vi "Set Echo Trigger Mode [ETM].vi"(7 "Micropulse # In":i32, 8 "error in (no error)":errorcluster, 9 "ETM Mode":T1, 11 "Test Number":u32) -> (0 "error out":errorcluster, 5 "Micropulse # Out":i32)   [LabVIEW 2026, in "MicroPulse_Driver.lvlib"]
doc: "Selects/deselects Interface Echo Trigger Modes, sometimes referred to as immersion testing with echo start. There several modes, one for calibration in conventional tests, one for echo trigger inspection in conventional/Phased Array tests and one for echo gate inspection in FMC tests. In echo trigger modes the echo gate is specified by the EGT(S) command and the inspection gate by the IGT(S) command. The trigger threshold level of the interface echo is set by the EUPL command for conventional tests and the EPL(S) command for Phased Array tests.\n\nMode = 0 : Normal triggering. (Default)\nMode = 1 : Display mode forms part of the calibration for conventional tests. Only the ‘Echo Gate’ is displayed allowing precise adjustment via the ‘EGT’ command.\n\nMode = 2 : Echo Trigger Mode for conventional tests. If a signal above the EUPL (is detected within the echo gate (EGT), MicroPulse processes the part of the signal derived from the IGT Parameters taken relative to the point in the echo gate where the signal breaks the EUPL.\n\nMode = 3 : For FMC Tests (AMP modes 13):\nEcho Trigger Mode for FMC tests If a signal above the EPL is detected within the echo gate (EGT), MicroPulse processes the part of the signal derived from the IGT Parameters taken relative to the point in the echo gate where the signal breaks the EPL. This happens independently on each receive channel used in the law. The data messages use a universal header format to accommodate the extra information required in this mode. For details on FMC mode interface echo see Appendix 6.5\nFor Multi-gate Tests (AMP modes 31 & 32):\nThe system performs interface echo mode and also output an Ascan that is referenced to the initial trigger. The interface echo range is now reported. It is now possible to set up an interface trigger gate, 4 hardware peak detection gates and 1 Ascan data gate on the same test. The interface echo range is output in an EGT range message (see Output Messages section)\n\nMode = 4 : Reserved\n\nMode = 5 : Echo Trigger Mode for Phased Array tests where a channel a contained within the focal law is specified as the interface trigger channel. The trigger channel must be contained within the focal law of the test. If a new focal law is applied to a test then the ETM mode is set back to 0, so the ETM mode (and therefore the trigger channel) must be resent. The interface echo range is output in an EGT range message (see Output messages section).\n\nParameters:\n<Tn> : Test number. An integer value from 0 to the maximum number of tests (default maximum is 1279 tests).\nTn = 0 for all conventional tests. If the S extension is used it applies to all tests in the sweep number specified: 1-32, 0 = all sweeps.\n\n<Mode> : \n0=Echo Trigger Mode ‘OFF’ (Default).\n1=Use Echo Trigger Gate (Conventional test only).\n2=Echo Trigger Mode ‘ON’ (Conventional/ Phased Array test).\n3=Echo Trigger Mode ‘ON’ (FMC test)/ Multi-gate with Ascan.\n5=Echo Trigger Mode ‘ON’ Phased Array channel trigger\n\n[Test No/CH] :\nUsed modes 2 and 5. In mode 2 it specifies a trigger test (256 - max test number), whilst in mode 5 it specifies a trigger channel (1 -128, but within the focal law)\n\nExample 1: \nETM 3 1 : Set test 3 to echo trigger display mode.\nETM 3 200 300 : Adjust interface echo monitor gate.\nETM 3 2 : Set test 3 to echo trigger mode.\n\nExample 2:\nAMP 256 32 : Set test amp mode to multi-gate\nEGT 256 1000 2000 : Set the interface trigger gate\nEPL 256 100 : Set the interface trigger gate threshold\nIGT 256 0 5000 : Set the interface trigger inspection gate\nETM 256 5 1 : Set the test to interface trigger on element 1\n\nNote 1:\nETM mode 2 can be used for phased array tests in non-FMC applications. For phased array tests the echo gate functions differently to conventional tests. For a Phased array test the user can specify another test (and therefore possibly another focal law) as the interface echo test. This test then triggers the inspection test relative to an interface echo found. The test to be used as the interface echo test is specified by using a third parameter on the ETM command.\nMode “ETM X 1” is not valid for phased array tests. The interface echo test can simply be displayed if required.\nDelay (DLY) and trim (TRM) are still used in echo gate mode for phased array tests. These parameters should normally be set to 0.\n\nNote 2:\nThe selection of an ETM mode for a test will clear any averaging setup on the test.\n\nNote 3:\nBy default, in ETM modes 3 and 5 the range of the interface echo is reported with an EGT Range message. To turn off this reporting use the ECON third parameter."
uses:
  MicroPulse_Driver.lvlib
  Data/Datatypes/MP - echo gate mode.ctl
  Private/MP-Registry Action-Enum.ctl
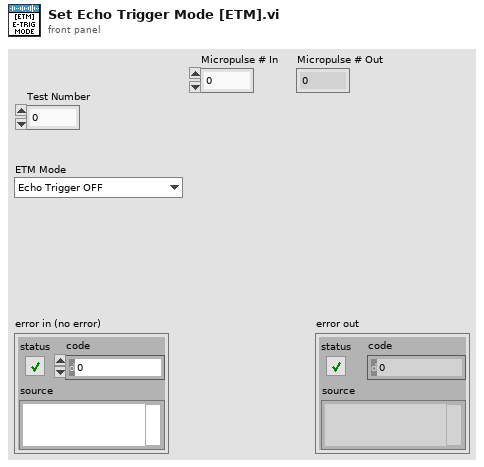
[diagram p1: front panel]
types:
  T1 = typedef "MicroPulse_Driver.lvlib/MP - echo gate mode.ctl" = enum16{"Echo Trigger OFF", "Echo Gate Display Mode", "Echo Trigger ON", "Multi Gate or FMC Mode", "Reserved", "PA - Echo Trigger ON"}
  T2 = typedef "MicroPulse_Driver.lvlib/MP-Registry Action-Enum.ctl" = enum16{"Read", "Add Test", "Add Command", "Add Gate Command", "Add Encoder Command", "Clear Command  List", "Set Registry", "Set System Details", "Set DOF", "Set Velocity", "Disable Asynch Reads", "Enable Asynch Reads", "Add Connection", "Disconnect", "Shutdown"}
  T3 = typedef "MicroPulse_Driver.lvlib/TCP config.ctl" = cluster{"Connection ID":refnum<k5>, "IP address":string, "host port":u16, "OC timeout":i32, "Read timeout":i32, "Write timeout":i32}
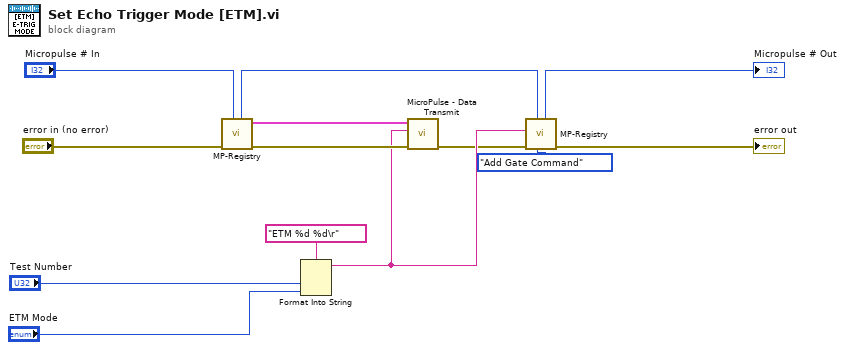
[diagram p0: block diagram]
diagram:
  n1 = call "MP-Registry.vi"("Micropulse # In"="Micropulse # In", "error in (no error)"="error in (no error)") -> ("error out"=w9:errorcluster, "TCP config"=w8:T3, "Micropulse # Out"=w4:i32)  [unwired: 6 in, 1 out]
  n2 = Format Into String(format string="ETM %d %d\r", "Test Number", "ETM Mode") -> (resulting string=w7:string)  [unwired: 2 in, 1 out]
  n3 = call "MicroPulse - Data Transmit.vi"("error in (no error)"=w9, "data"=w7, "TCP config"=w8) -> ("error out"=w5:errorcluster)  [unwired: 6 in, 2 out]
  n4 = call "MP-Registry.vi"("Action"=MP-Registry_Action-Enum."Add Gate Command", "Micropulse # In"=w4, "error in (no error)"=w5, "Data in"=w7) -> ("error out"=→"error out":errorcluster, "Micropulse # Out"=→"Micropulse # Out":i32)  [unwired: 4 in, 2 out]
